vi "单路通断器（VAR).vi"(1 "默认值":variant, 2 "直通？":bool=TRUE, 3 "X_In":variant) -> (0 "X_Out":variant)   [LabVIEW 2012]
doc: "功能：\n\n返回一个枚举，表明输入数的范围，用于三段比较。\n\n\nCSXCS_366创建。"
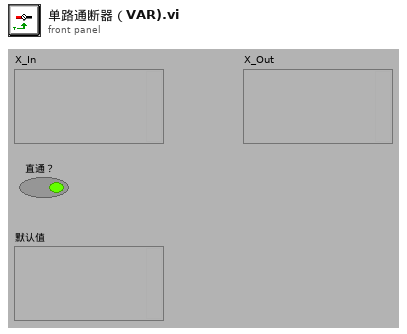
[diagram p1: front panel]
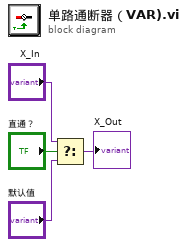
[diagram p0: block diagram]
diagram:
  n1 = Select(t="X_In", s="直通？", f="默认值") -> (s? t:f=→"X_Out":variant)
